vi "复材超声C扫缺陷分析评定软件-修改中.vi"() -> ()   [LabVIEW 2018]
doc: "使用该模板构建用户界面事件处理设计模式。将模板应用于对话框及其它用户界面。用户也可创建并执行VI可按照与用户界面事件相同方式处理的用户定义事件。"
uses:
  <vilib>/Utility/NIReport.llb/Report Type.ctl
  <vilib>/addons/_office/_exclsub.llb/font.ctl
  <vilib>/addons/_office/word.llb/Word Easy Table (str).vi
  <vilib>/Utility/NIReport.llb/NI_report.lvclass
  <vilib>/vision/NI_Vision_Development_Module.lvlib
  <vilib>/Utility/NIReport.llb/NI_ReportGenerationCore.lvlib
  <vilib>/addons/_office/NI_ReportGenerationToolkit.lvlib
panel:
  out "标注后的图片路径":path
  out "弥散类检测结果合并":string[][](table)
  out "分层类检测结果合并":string[][](table)
  out "反射图原始路径":path
  out "穿透图原始路径":path
  out "弥散类检测结果":string[][](table)
  out "分层类检测结果":string[][](table)
  out "部位信息":string[](array[string])=["", "34.500000", "32.500000", "1121", "34", "54.955926", "分层类", "不合格", ""]
  out "连接的字符串":string
  in  "完成标注":bool caption="定量分析"
  out "框数":dbl
  in  "Operation":enum16{"overlay rectangle"}(ring)
  out "ROI左上角坐标":cluster{i32, i32}
  out "自定义字体":T1={"Desired Font (Application)"=enum."Application Font", "[User-specified Font]"={"Font Name"="", "Size"=12, "Strikeout?"=FALSE, "Italic?"=FALSE, "Underline?"=FALSE, "Outline?"=FALSE, "Shadow?"=FALSE, "Bold?"=FALSE, "Rotation Angle"=0.0}, "Horizontal Alignment"=0, "Vertical Alignment"=0} {"Horizontal Alignment" items=["Left", "Center", "Right"]; "Vertical Alignment" items=["Bottom", "Top", "Baseline"]}
  out "标注图ROI2Mask":T2(plugin-control)
  out "透射图最大灰度值":sgl
  out "反射图最大灰度值":sgl
  out "反射图灰度表":u32[](graph)
  out "透射图灰度表":u32[](graph)
  out "总面积":i32
  out "框组":T3(array[cluster])
  out "质量等级":string
  in  "导入反射图":bool caption="导入图片"
  out "灰度阈值":dbl
  in  "stop":bool caption="停止"
  in  "导入穿透图":bool caption="导入图片"
  in  "图像预处理":bool
  in  "自定义色彩":bool
  in  "缺陷标注":bool caption="定量分析"
  in  "查看标注":bool caption="辅助定性分析"
  in  "生成评定结果":bool caption="生成原始记录"
  in  "?":enum32{"穿透图", "反射图"}(tab)
  out "穿透图":T2(plugin-control)
  out "反射图":T2(plugin-control)
  out "产品规格":cluster{"产品长度（周长）（mm）":dbl, "产品宽度（母线长）（mm）":dbl}
  out "图像分辨率":T4
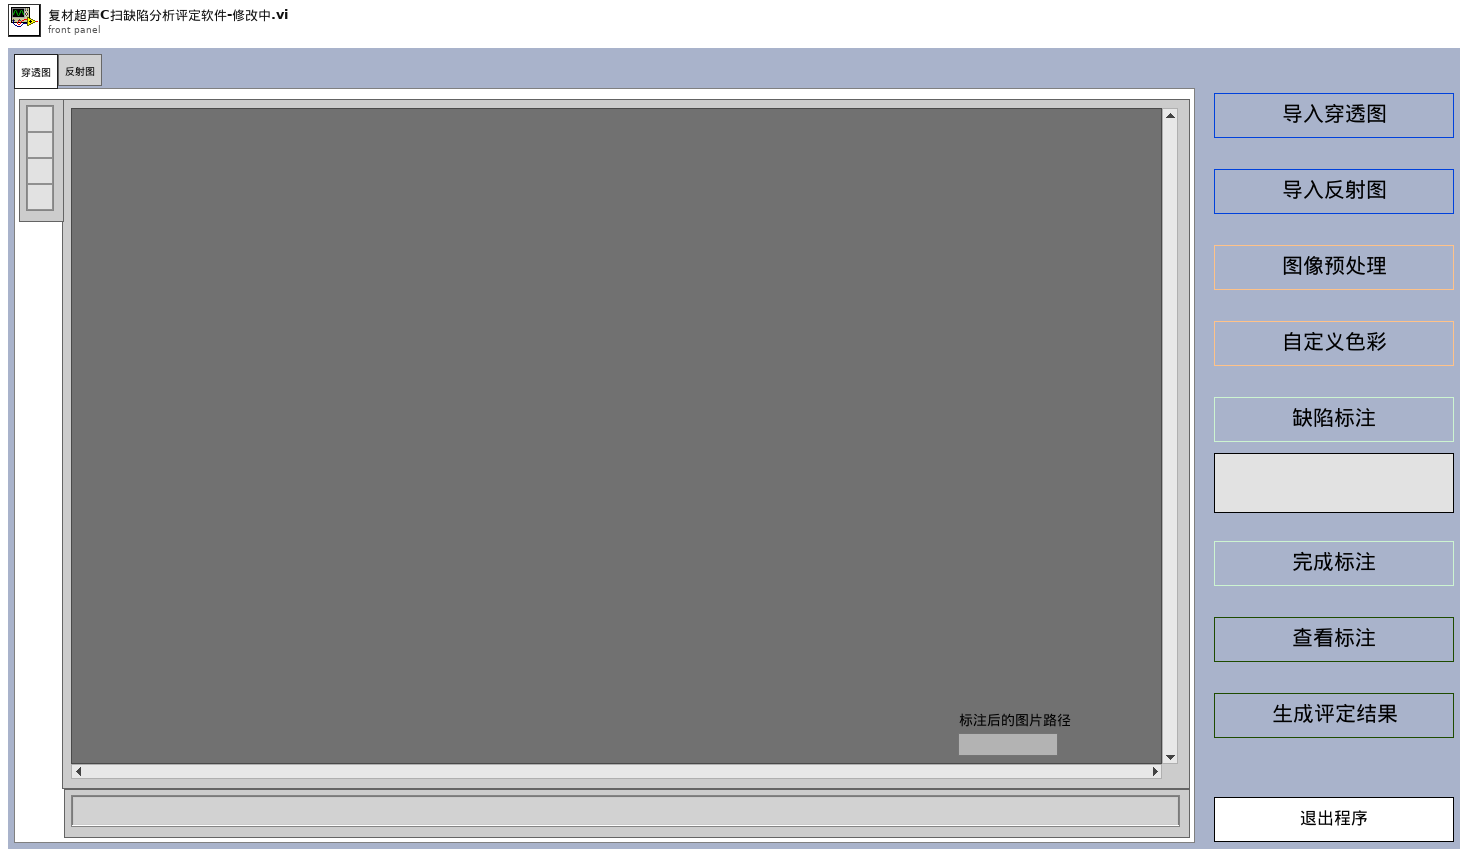
[diagram p1: front panel]
types:
  T1 = cluster{"Desired Font (Application)":enum16{"User-specified Font", "Application Font", "System Font", "Dialog Font"}, "[User-specified Font]":cluster{"Font Name":string, "Size":i16, "Strikeout?":bool, "Italic?":bool, "Underline?":bool, "Outline?":bool, "Shadow?":bool, "Bold?":bool, "Rotation Angle":dbl}, "Horizontal Alignment":i16, "Vertical Alignment":i16}
  T2 = typedef "IMAQ Image.ctl" = refnum<image>
  T3 = cluster{"Global Rectangle":i32[], "Contours":cluster{"Contour Type":u32, "ROI Type":u32, "Points":i32[]}[]}[]
  T4 = cluster{"图像X向分辨率（mm/像素）":dbl, "图像Y向分辨率（mm/像素）":dbl}
  T5 = cluster{"Zoom Tool":bool, "Selection Tool":bool, "Pan Tool":bool, "Point Tool":bool, "Line Tool":bool, "Rectangle Tool":bool, "Rotated Rectangle Tool":bool, "Polyline Tool":bool, "Polygon Tool":bool, "Freehand Tool":bool, "Closed Freehand Tool":bool, "Ellipse Tool":bool, "Annulus Tool":bool}
  T6 = enum32{"Invalid", "Standard", "Closed", "Hidden", "Minimized", "Maximized"}
  T7 = enum32{"Linear", "Log", "Exp", "Square", "Square root", "Power X", "Power 1/X"}
  T8 = enum32{"Gray", "Binary", "Gradient", "Rainbow", "Temperature"}
  T9 = typedef "NI_ReportGenerationToolkit.lvlib/font.ctl" = cluster{"font name":string, "font size":dbl, "bold":u16, "italic":u16, "underline":u16, "strike through":u16, "font color":u32}
  T10 = enum16{"maximized", "minimized", "normal", "no change"}
  T11 = typedef "NI_ReportGenerationCore.lvlib/Report Type.ctl" = enum16{"HTML", "Word", "Excel"}
  T12 = typedef "Image Type" = u32
  T13 = cluster{"Red (or Hue) value":u8, "Green (or Sat) value":u8, "Blue (or Light or Val) value":u8}[]
  T14 = cluster{"histogram":u32[], "Minimal Value":sgl, "Maximal Value":sgl, "Starting Value":sgl, "Interval Width":sgl, "Mean Value":sgl, "Standard  Variation":sgl, "Area (pixels)":i32}
  T15 = cluster{"Global Rectangle":i32[], "Contours":cluster{"Contour Type":u32, "ROI Type":u32, "Points":i32[]}[]}
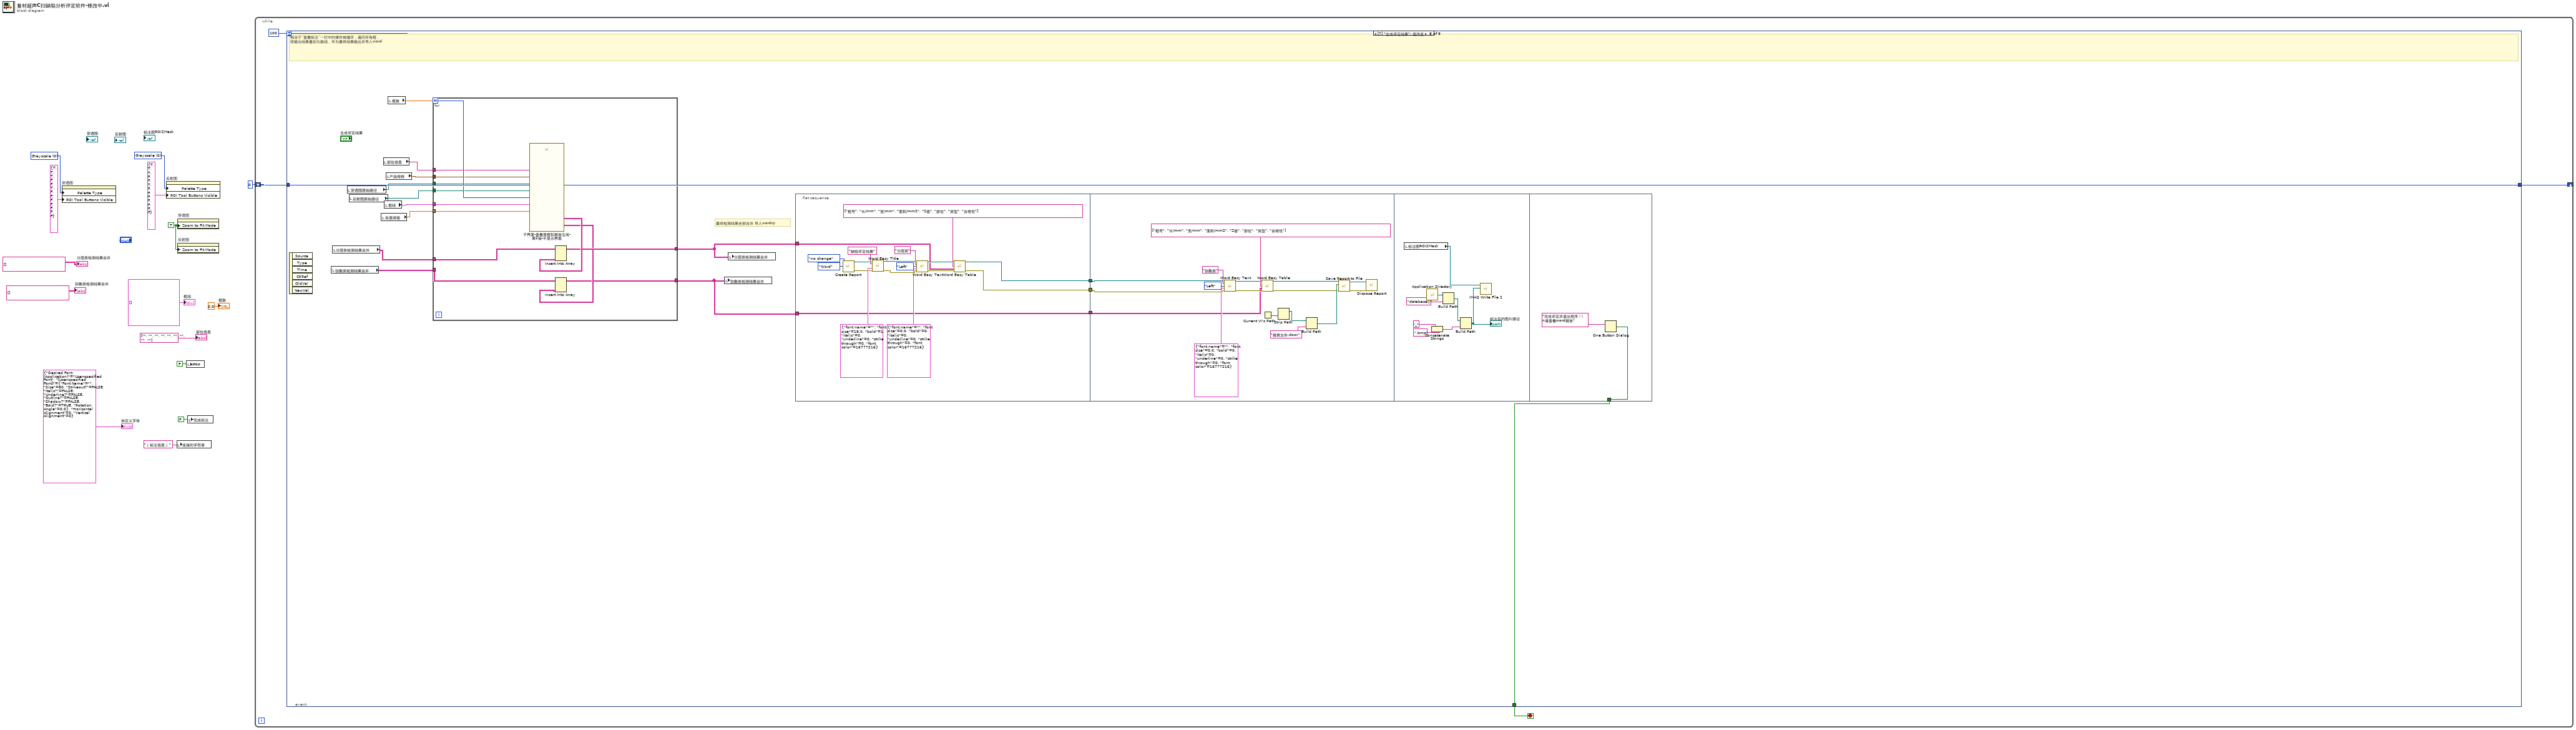
[diagram p0: block diagram]
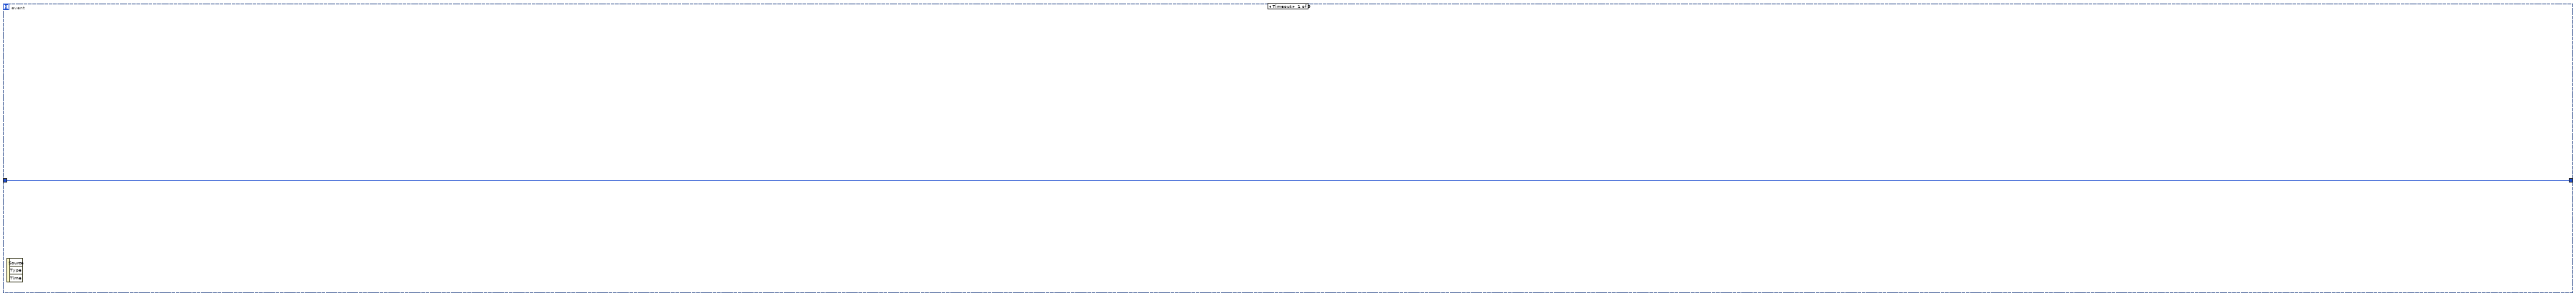
[diagram p2: hidden frame]
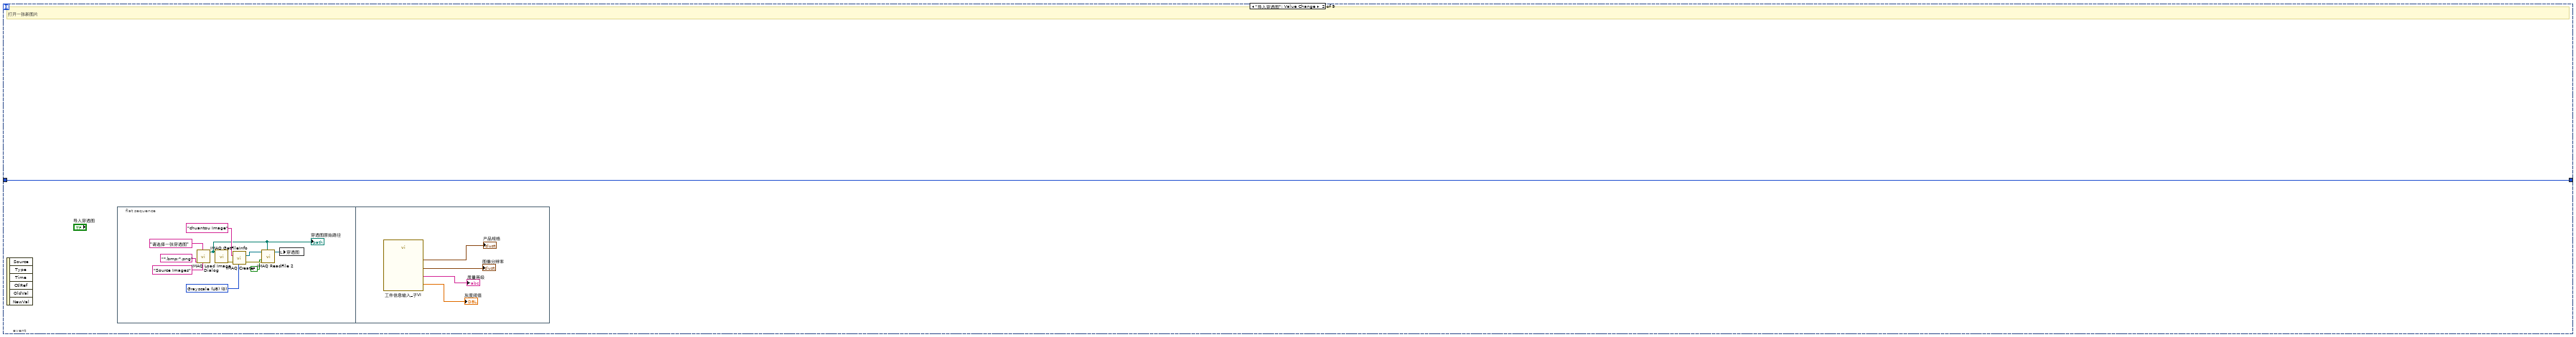
[diagram p3: hidden frame]
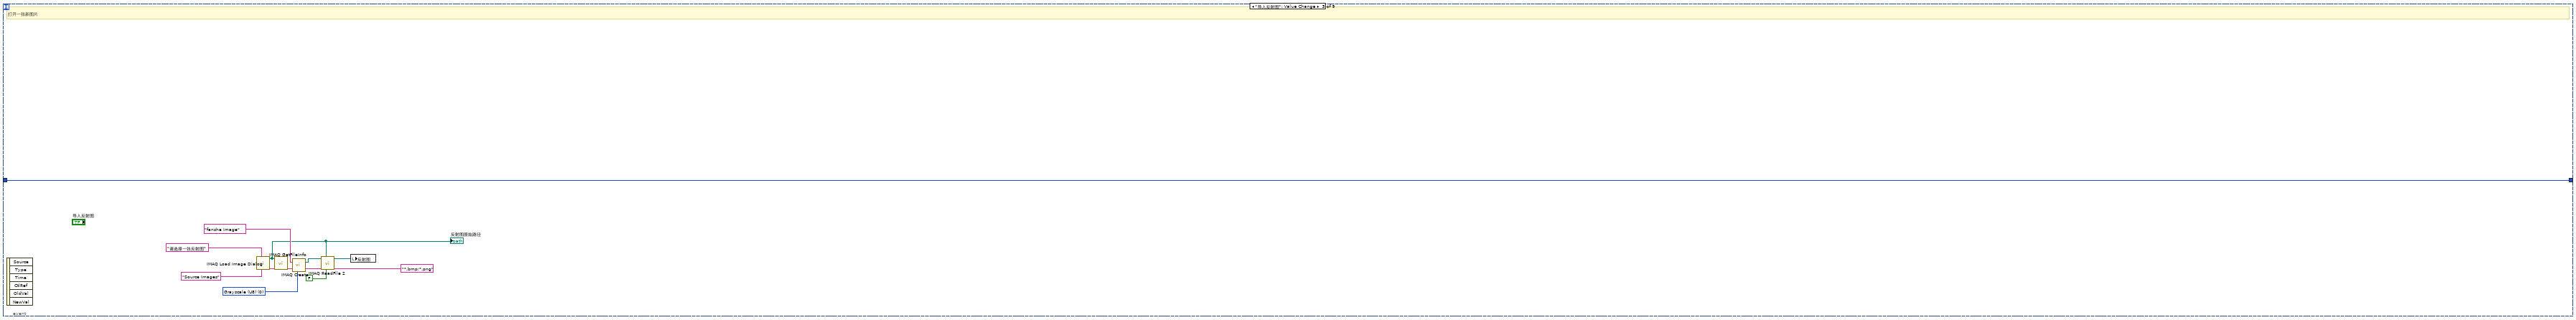
[diagram p4: hidden frame]
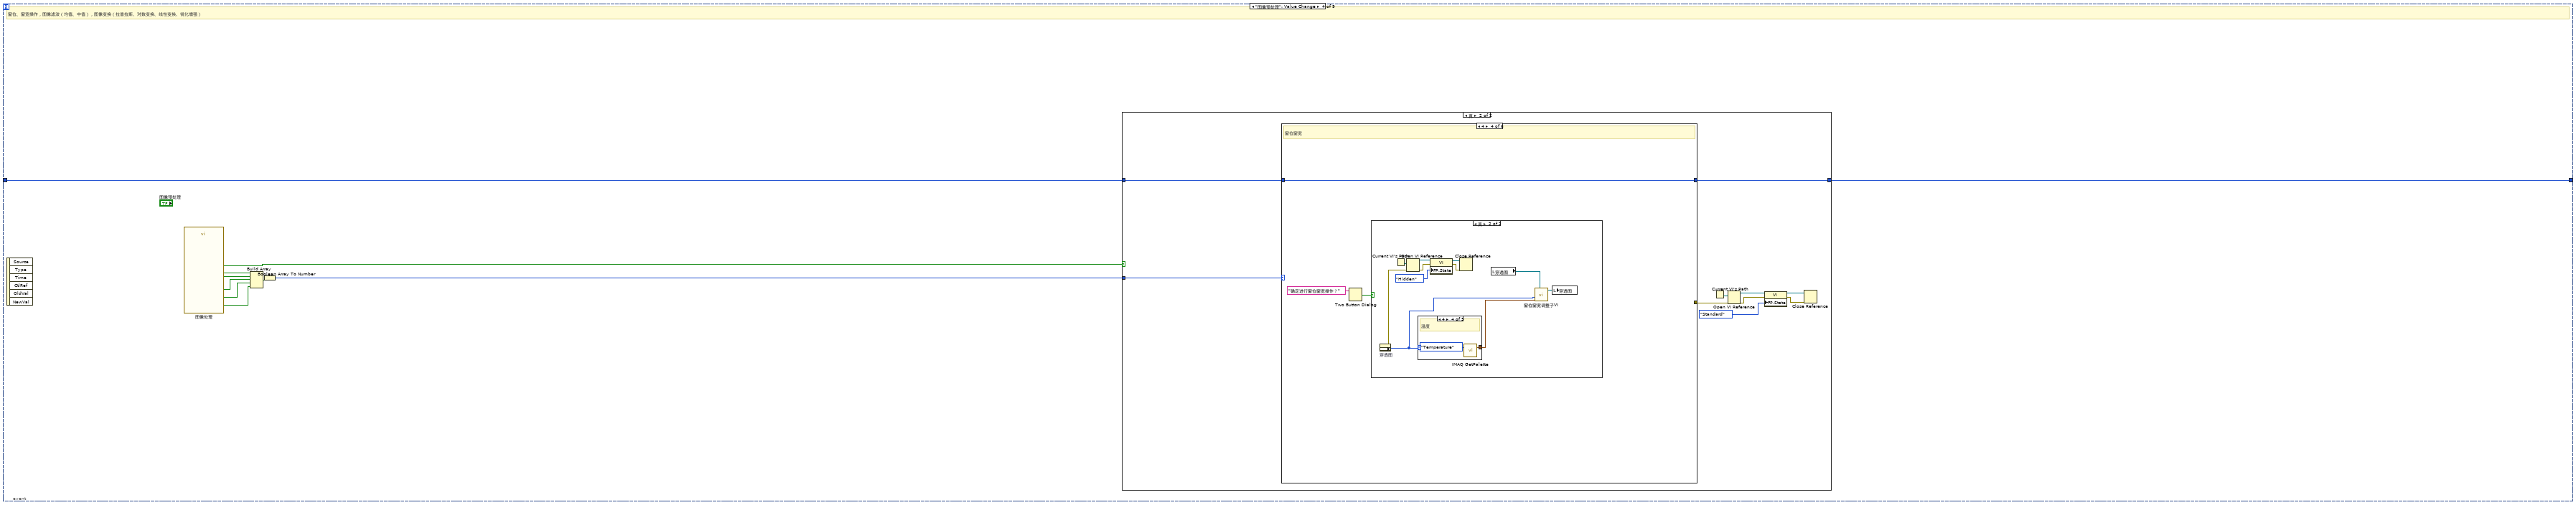
[diagram p5: hidden frame]
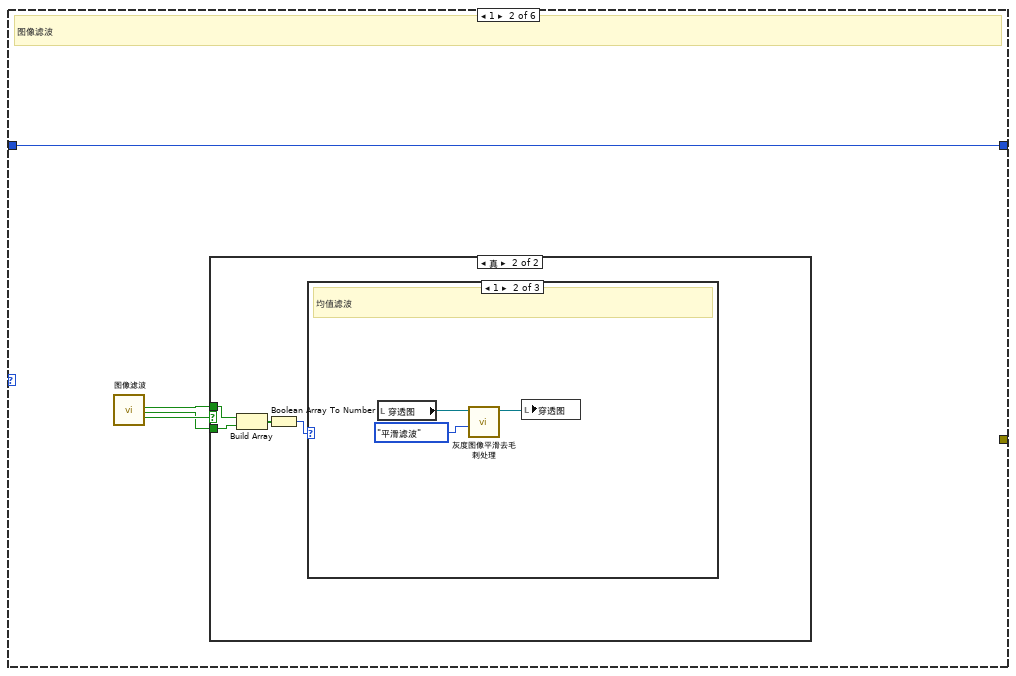
[diagram p8: hidden frame]
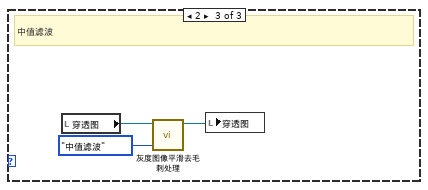
[diagram p11: hidden frame]
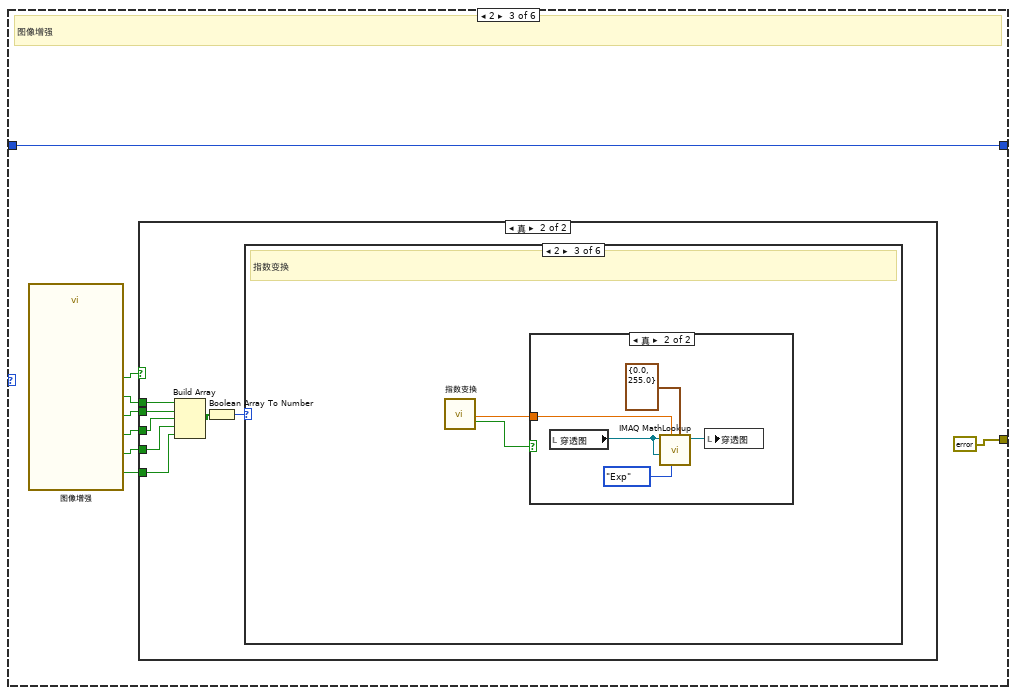
[diagram p12: hidden frame]
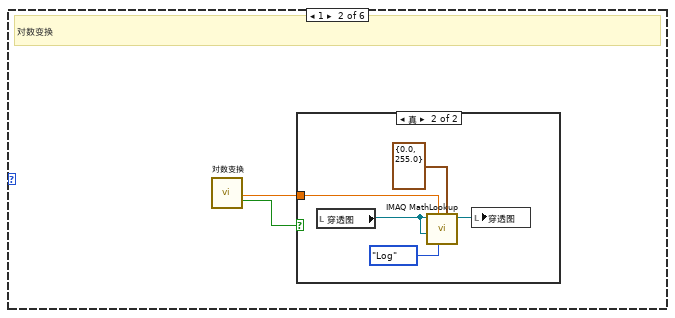
[diagram p15: hidden frame]
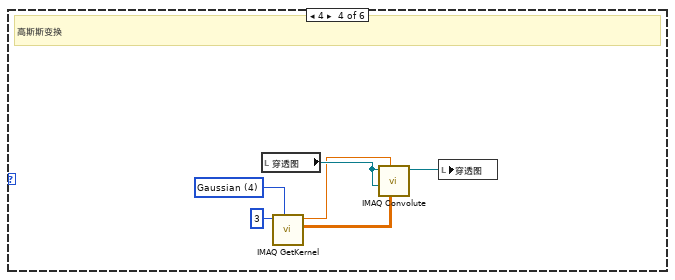
[diagram p18: hidden frame]
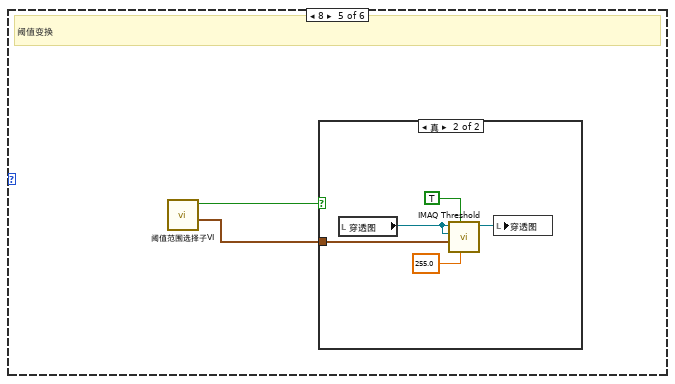
[diagram p19: hidden frame]
diagram:
  w5 = u32 0 items=["Grayscale", "Binary", "Gradient", "Rainbow", "Temperature", "User Defined", "Binary 16 Bit", "Gradient 16 Bit", "Rainbow 16 Bit", "Temperature 16 Bit", "User Defined 16 Bit"] ("Palette:Palette Type")
  w11 = TRUE ("Zoom to Fit Mode")
  w14 = u32 0 items=["Grayscale", "Binary", "Gradient", "Rainbow", "Temperature", "User Defined", "Binary 16 Bit", "Gradient 16 Bit", "Rainbow 16 Bit", "Temperature 16 Bit", "User Defined 16 Bit"] ("Palette:Palette Type")
  n1 = property on="穿透图" class="ImageControl"("Palette Type"=w14, "ROI Tool Buttons Visible"=T5 {"Zoom Tool"=TRUE, "Selection Tool"=TRUE, "Pan Tool"=TRUE, "Point Tool"=FALSE, "Line Tool"=FALSE, "Rectangle Tool"=TRUE, "Rotated Rectangle Tool"=FALSE, "Polyline Tool"=FALSE, "Polygon Tool"=FALSE, "Freehand Tool"=FALSE, "Closed Freehand Tool"=FALSE, "Ellipse Tool"=FALSE, "Annulus Tool"=FALSE} ("ROI Tool Buttons Visible:All Elements")) -> ()  [unwired: 2 in, 2 out]
  n2 = property on="反射图" class="ImageControl"("Palette Type"=w5, "ROI Tool Buttons Visible"=T5 {"Zoom Tool"=TRUE, "Selection Tool"=TRUE, "Pan Tool"=TRUE, "Point Tool"=FALSE, "Line Tool"=FALSE, "Rectangle Tool"=TRUE, "Rotated Rectangle Tool"=FALSE, "Polyline Tool"=FALSE, "Polygon Tool"=FALSE, "Freehand Tool"=FALSE, "Closed Freehand Tool"=FALSE, "Ellipse Tool"=FALSE, "Annulus Tool"=FALSE} ("ROI Tool Buttons Visible:All Elements")) -> ()  [unwired: 2 in, 2 out]
  n3 = local write "连接的字符串"("（标注信息）" ("连接的字符串")) -> ()
  n4 = property on="穿透图" class="ImageControl"("Zoom to Fit Mode"=w11) -> ()  [unwired: 2 in, 2 out]
  n5 = property on="反射图" class="ImageControl"("Zoom to Fit Mode"=w11) -> ()  [unwired: 2 in, 2 out]
  n6 = local write "stop"(FALSE ("stop")) -> ()
  n7 = local write "完成标注"(FALSE ("完成标注")) -> ()
  n8 = while {
    shift-right: [w16] -> _
    shift-left: 0 -> [w17]
    stop <- w19 stop-if-true
    n9 = event shown="[7] \"生成评定结果\": 值改变" {
      selector: _ -> [_ _ _ _ _ _ _ _ _]
      dyn-events: _ -> [_ _ _ _ _ _ _ _ _]
      timeout: 100 -> [_ _ _ _ _ _ _ _ _]
      tunnel: [_ _ _ _ _ _ _ w396 w471] -> w19
      tunnel: w17 -> [w20 w21 w48 w50 w188 _ _ w411 _]
      tunnel: [w20 w21 w48 w49 w188 _ _ w411 0] -> w16
      event Timeout {
        n10 = event-data() -> ()  [unwired: 1 in, 3 out]
      }
      event "导入穿透图": Value Change {
        # "打开一张新图片"
        n11 = event-data() -> ()  [unwired: 1 in, 6 out]
        n12 = flat-sequence {
          frame #0 {
            w24 = T12 0 items=["Grayscale (U8)", "Grayscale (I16)", "Grayscale (SGL)", "Complex (CSG)", "RGB (U32)", "HSL (U32)", "RGB (U64)", "Grayscale (U16)"] ("Image Type")
            n13 = call "IMAQ Load Image Dialog"("Pattern Label"="Source Images", "Prompt"="请选择一张穿透图" ("prompt"), "Pattern"="*.bmp;*.png") -> ("Path"=w22:path)  [unwired: 6 in, 2 out]
            "穿透图原始路径" <- w22
            n14 = call "IMAQ GetFileInfo"("File Path"=w22) -> ("error out"=w27:errorcluster)  [unwired: 4 in, 6 out]
            n15 = call "IMAQ Create"("Image Name"="chuantou Image", "Image Type"=w24, "error in (no error)"=w27) -> ("New Image"=w28:T2, "error out"=w29:errorcluster)  [unwired: 2 in]
            n16 = call "IMAQ ReadFile 2"("Use File Path Image Type"=FALSE, "File Path"=w22, "error in (no error)"=w29, "Image"=w28) -> ("Image Out"=w23:T2)  [unwired: 3 in, 4 out]
            n17 = local write "穿透图"(w23) -> ()
          }
          frame #1 {
            n18 = call "工件信息输入_子VI.vi"() -> ("质量等级"=→"质量等级":string, "灰度阈值"=→"灰度阈值":dbl, "产品规格"=→"产品规格":cluster{"产品长度（周长）（mm）":dbl, "产品宽度（母线长）（mm）":dbl}, "图像分辨率"=→"图像分辨率":T4)  [unwired: 7 in]
          }
        }
      }
      event "导入反射图": Value Change {
        w39 = T12 0 items=["Grayscale (U8)", "Grayscale (I16)", "Grayscale (SGL)", "Complex (CSG)", "RGB (U32)", "HSL (U32)", "RGB (U64)", "Grayscale (U16)"] ("Image Type")
        # "打开一张新图片"
        n19 = event-data() -> ()  [unwired: 1 in, 6 out]
        n20 = call "IMAQ Load Image Dialog"("Pattern Label"="Source Images", "Prompt"="请选择一张反射图" ("prompt"), "Pattern"="*.bmp;*.png") -> ("Path"=w37:path)  [unwired: 6 in, 2 out]
        "反射图原始路径" <- w37
        n21 = call "IMAQ GetFileInfo"("File Path"=w37) -> ("error out"=w42:errorcluster)  [unwired: 4 in, 6 out]
        n22 = call "IMAQ Create"("Image Name"="fanshe Image", "Image Type"=w39, "error in (no error)"=w42) -> ("New Image"=w43:T2, "error out"=w44:errorcluster)  [unwired: 2 in]
        n23 = call "IMAQ ReadFile 2"("Use File Path Image Type"=FALSE, "File Path"=w37, "error in (no error)"=w44, "Image"=w43) -> ("Image Out"=w38:T2)  [unwired: 3 in, 4 out]
        n24 = local write "反射图"(w38) -> ()
      }
      event "图像预处理": Value Change {
        # "窗位、窗宽操作，图像滤波（均值、中值），图像变换（拉普拉斯、对数变换、线性变换、锐化增强）"
        n25 = event-data() -> ()  [unwired: 1 in, 6 out]
        n26 = call "图像处理"() -> ("撤销图像处理"=w51:bool, "线性灰度值测量"=w52:bool, "窗位窗宽"=w57:bool, "图像增强"=w53:bool, "图像滤波"=w58:bool, "确定"=w54:bool)  [unwired: 13 in, 1 out]
        n27 = Build Array(w58, w53, w57, w52, w51) -> (w56:bool[])
        n28 = Boolean Array To Number(Boolean array=w56) -> (number=w55:u32)
        n29 = case shown="真" w54 {
          tunnel: w55 -> [_ w69]
          tunnel: w50 -> [w59 w61]
          tunnel: [w59 w60] -> w49
          frame False {
          }
          frame True {
            n30 = case shown="4" w69 {
              tunnel: [_ _ errorcluster {"status"=FALSE, "code"=0, "source"=""} ("错误输入（无错误）") _ _ _] -> w62
              tunnel: w61 -> [w70 w71 w85 w134 w157 w179]
              tunnel: [w70 w71 w85 w134 w157 w179] -> w60
              frame 0, Default {
              }
              frame 1 {
                # "图像滤波"
                n31 = call "图像滤波"() -> ("均值滤波"=w73:bool, "中值滤波"=w72:bool, "确定"=w74:bool)  [unwired: 16 in, 1 out]
                n32 = case shown="真" w74 {
                  tunnel: w73 -> [_ w77]
                  tunnel: w72 -> [_ w76]
                  frame False {
                  }
                  frame True {
                    n33 = Build Array(w77, w76) -> (w78:bool[])
                    n34 = Boolean Array To Number(Boolean array=w78) -> (number=w75:u32)
                    n35 = case shown="1" w75 {
                      frame 0, Default {
                      }
                      frame 1 {
                        # "均值滤波"
                        n36 = local read "穿透图"() -> (w81:T2)
                        n37 = call "灰度图像平滑去毛刺处理.vi"("滤波方法选择"=enum16{"中值滤波", "平滑滤波"}."平滑滤波", "Image"=w81) -> ("Image Out"=w80:T2)  [unwired: 9 in]
                        n38 = local write "穿透图"(w80) -> ()
                      }
                      frame 2 {
                        # "中值滤波"
                        n39 = local read "穿透图"() -> (w84:T2)
                        n40 = call "灰度图像平滑去毛刺处理.vi"("滤波方法选择"=enum16{"中值滤波", "平滑滤波"}."中值滤波", "Image"=w84) -> ("Image Out"=w83:T2)  [unwired: 9 in]
                        n41 = local write "穿透图"(w83) -> ()
                      }
                    }
                  }
                }
              }
              frame 2 {
                # "图像增强"
                n42 = call "图像增强"() -> ("幂变换"=w87:bool, "阈值变换"=w88:bool, "高斯变换"=w89:bool, "指数变换"=w90:bool, "对数变换"=w91:bool, "确定"=w92:bool)  [unwired: 13 in, 1 out]
                n43 = case shown="真" w92 {
                  tunnel: w91 -> [_ w97]
                  tunnel: w90 -> [_ w96]
                  tunnel: w89 -> [_ w95]
                  tunnel: w88 -> [_ w94]
                  tunnel: w87 -> [_ w93]
                  frame False {
                  }
                  frame True {
                    n44 = Build Array(w97, w96, w95, w94, w93) -> (w99:bool[])
                    n45 = Boolean Array To Number(Boolean array=w99) -> (number=w98:u32)
                    n46 = case shown="2" w98 {
                      frame 0, Default {
                      }
                      frame 1 {
                        # "对数变换"
                        n47 = call "对数变换"() -> ("变换系数K"=w100:dbl, "确定"=w101:bool)  [unwired: 17 in, 1 out]
                        n48 = case shown="真" w101 {
                          tunnel: w100 -> [_ w102]
                          frame False {
                          }
                          frame True {
                            n49 = local read "穿透图"() -> (w106:T2)
                            n50 = call "IMAQ MathLookup"("Range"=cluster{"Minimum":sgl, "Maximum":sgl} {"Minimum"=0.0, "Maximum"=255.0}, "Operator"=T7."Log", "X Value"=w102, "Image Dst"=w106, "Image Src"=w106) -> ("Image Dst Out"=w104:T2)  [unwired: 5 in, 1 out]
                            n51 = local write "穿透图"(w104) -> ()
                          }
                        }
                      }
                      frame 2 {
                        # "指数变换"
                        n52 = call "指数变换"() -> ("变换系数K"=w107:dbl, "确定"=w108:bool)  [unwired: 17 in, 1 out]
                        n53 = case shown="真" w108 {
                          tunnel: w107 -> [_ w109]
                          frame False {
                          }
                          frame True {
                            n54 = local read "穿透图"() -> (w113:T2)
                            n55 = call "IMAQ MathLookup"("Range"=cluster{"Minimum":sgl, "Maximum":sgl} {"Minimum"=0.0, "Maximum"=255.0}, "Operator"=T7."Exp", "X Value"=w109, "Image Dst"=w113, "Image Src"=w113) -> ("Image Dst Out"=w111:T2)  [unwired: 5 in, 1 out]
                            n56 = local write "穿透图"(w111) -> ()
                          }
                        }
                      }
                      frame 4 {
                        w119 = u16 4 items=["Gradient"=1, "Laplacian"=2, "Smoothing"=3, "Gaussian"=4] ("Kernel Family")
                        # "高斯斯变换"
                        n57 = local read "穿透图"() -> (w116:T2)
                        n58 = call "IMAQ GetKernel"("Kernel Family"=w119, "Kernel Size (3,5,...)"=3) -> ("Kernel"=w117:sgl[][], "Divider"=w114:sgl)  [unwired: 6 in, 2 out]
                        n59 = call "IMAQ Convolute"("Kernel"=w117, "Divider (kernel sum)"=w114, "Image Dst"=w116, "Image Src"=w116) -> ("Image Dst Out"=w115:T2)  [unwired: 6 in, 1 out]
                        n60 = local write "穿透图"(w115) -> ()
                      }
                      frame 8 {
                        # "阈值变换"
                        n61 = call "阈值范围选择子VI.vi"() -> ("阈值范围"=w120:cluster{"Lower value":sgl, "Upper value":sgl}, "确定执行"=w121:bool)  [unwired: 10 in]
                        n62 = case shown="真" w121 {
                          tunnel: w120 -> [_ w123]
                          frame False {
                          }
                          frame True {
                            n63 = local read "穿透图"() -> (w126:T2)
                            n64 = call "IMAQ Threshold"("Replace Value"=sgl 255.0, "Keep/Replace Value (Replace)"=TRUE, "Range"=w123, "Image Dst"=w126, "Image Src"=w126) -> ("Image Dst Out"=w125:T2)  [unwired: 5 in, 1 out]
                            n65 = local write "穿透图"(w125) -> ()
                          }
                        }
                      }
                      frame 16 {
                        # "幂变换"
                        n66 = call "幂变换"() -> ("变换系数K"=w127:dbl, "确定"=w128:bool)  [unwired: 17 in, 1 out]
                        n67 = case shown="真" w128 {
                          tunnel: w127 -> [_ w129]
                          frame False {
                          }
                          frame True {
                            n68 = local read "穿透图"() -> (w133:T2)
                            n69 = call "IMAQ MathLookup"("Range"=cluster{"Minimum":sgl, "Maximum":sgl} {"Minimum"=0.0, "Maximum"=255.0}, "Operator"=T7."Power 1/X", "X Value"=w129, "Image Dst"=w133, "Image Src"=w133) -> ("Image Dst Out"=w131:T2)  [unwired: 5 in, 1 out]
                            n70 = local write "穿透图"(w131) -> ()
                          }
                        }
                      }
                    }
                  }
                }
              }
              frame 4 {
                # "窗位窗宽"
                n71 = Two Button Dialog(message="确定进行窗位窗宽操作？" ("消息")) -> (T button?=w136:bool)  [unwired: 2 in]
                n72 = case shown="真" w136 {
                  frame False {
                  }
                  frame True {
                    n73 = property on="穿透图" class="ImageControl"() -> (error out=w138:errorcluster, "Palette Type"=w145:u32)  [unwired: 2 in, 1 out]
                    n74 = Current VI's Path() -> (path=w140:path)
                    n75 = Open VI Reference(vi path=w140, error in (no error)=w138) -> (vi reference=w141:refnum<vi>, error out=w143:errorcluster)  [unwired: 4 in]
                    n76 = case shown="4" w145 {
                      tunnel: [w148 w150 w152 w154 w156] -> w146
                      frame 0, Default {
                        # "灰度"
                        n77 = call "IMAQ GetPalette"("Palette Number (gray)"=T8."Gray") -> ("Color Palette"=w148:cluster{"Red":u8, "Green":u8, "Blue":u8}[])  [unwired: 4 in, 1 out]
                      }
                      frame 2 {
                        # "梯度"
                        n78 = call "IMAQ GetPalette"("Palette Number (gray)"=T8."Gradient") -> ("Color Palette"=w150:cluster{"Red":u8, "Green":u8, "Blue":u8}[])  [unwired: 4 in, 1 out]
                      }
                      frame 3 {
                        # "彩虹"
                        n79 = call "IMAQ GetPalette"("Palette Number (gray)"=T8."Rainbow") -> ("Color Palette"=w152:cluster{"Red":u8, "Green":u8, "Blue":u8}[])  [unwired: 4 in, 1 out]
                      }
                      frame 4 {
                        # "温度"
                        n80 = call "IMAQ GetPalette"("Palette Number (gray)"=T8."Temperature") -> ("Color Palette"=w154:cluster{"Red":u8, "Green":u8, "Blue":u8}[])  [unwired: 4 in, 1 out]
                      }
                      frame 5 {
                        # "自定义"
                        n81 = property on="穿透图" class="ImageControl"() -> ("User Palette"=w156:cluster{"Red":u8, "Green":u8, "Blue":u8}[])  [unwired: 2 in, 2 out]
                      }
                    }
                    n82 = property class="VI"(reference=w141, error in=w143, "FP.State"=T6."Hidden" ("前面板窗口:状态")) -> (reference out=w142:refnum<vi>, error out=w144:errorcluster)
                    n83 = Close Reference(reference=w142, error in (no error)=w144) -> ()  [unwired: 1 out]
                    n84 = local read "穿透图"() -> (w137:T2)
                    n85 = call "窗位窗宽调整子VI.vi"("Image in"=w137, "Palette:User Palette"=w146, "Palette:Palette Type"=w145) -> ("Image out"=w147:T2)  [unwired: 8 in]
                    n86 = local write "穿透图"(w147) -> ()
                  }
                }
              }
              frame 8 {
                # "查看线灰度值曲线，用于精确测量"
                n87 = Current VI's Path() -> (path=w164:path)
                n88 = Open VI Reference(vi path=w164) -> (vi reference=w163:refnum<vi>, error out=w161:errorcluster)  [unwired: 5 in]
                n89 = property class="VI"(reference=w163, error in=w161, "FP.State"=T6."Hidden" ("前面板窗口:状态")) -> (reference out=w162:refnum<vi>, error out=w160:errorcluster)
                n90 = Close Reference(reference=w162, error in (no error)=w160) -> (error out=w158:errorcluster)
                n91 = case shown="无错误" w158 {
                  frame No Error {
                    n92 = property on="穿透图" class="ImageControl"() -> ("Palette Type"=w166:u32)  [unwired: 2 in, 2 out]
                    n93 = case shown="2" w166 {
                      tunnel: [w169 w171 w173 w175 w177] -> w165
                      frame 0, Default {
                        # "灰度"
                        n94 = call "IMAQ GetPalette"("Palette Number (gray)"=T8."Gray") -> ("Color Palette"=w169:cluster{"Red":u8, "Green":u8, "Blue":u8}[])  [unwired: 4 in, 1 out]
                      }
                      frame 2 {
                        # "梯度"
                        n95 = call "IMAQ GetPalette"("Palette Number (gray)"=T8."Gradient") -> ("Color Palette"=w171:cluster{"Red":u8, "Green":u8, "Blue":u8}[])  [unwired: 4 in, 1 out]
                      }
                      frame 3 {
                        # "彩虹"
                        n96 = call "IMAQ GetPalette"("Palette Number (gray)"=T8."Rainbow") -> ("Color Palette"=w173:cluster{"Red":u8, "Green":u8, "Blue":u8}[])  [unwired: 4 in, 1 out]
                      }
                      frame 4 {
                        # "温度"
                        n97 = call "IMAQ GetPalette"("Palette Number (gray)"=T8."Temperature") -> ("Color Palette"=w175:cluster{"Red":u8, "Green":u8, "Blue":u8}[])  [unwired: 4 in, 1 out]
                      }
                      frame 5 {
                        # "自定义"
                        n98 = property on="穿透图" class="ImageControl"() -> ("User Palette"=w177:cluster{"Red":u8, "Green":u8, "Blue":u8}[])  [unwired: 2 in, 2 out]
                      }
                    }
                    n99 = local read "穿透图"() -> (w168:T2)
                    n100 = local read "图像分辨率"() -> (w167:T4)
                    n101 = call "线性灰度值曲线查看子VI.vi"("Palette:User Palette"=w165, "图像分辨率"=w167, "Image"=w168) -> ()  [unwired: 9 in]
                  }
                  frame Error {
                  }
                }
              }
              frame 16 {
                # "撤销图像处理，恢复原图"
                n102 = call "IMAQ Create"("Image Name"="P1") -> ("New Image"=w178:T2)  [unwired: 4 in, 1 out]
                n103 = local write "穿透图"(w178) -> ()
              }
            }
            n104 = Current VI's Path() -> (path=w68:path)
            n105 = Open VI Reference(vi path=w68, error in (no error)=w62) -> (vi reference=w67:refnum<vi>, error out=w64:errorcluster)  [unwired: 4 in]
            n106 = property class="VI"(reference=w67, error in=w64, "FP.State"=T6."Standard" ("前面板窗口:状态")) -> (reference out=w65:refnum<vi>, error out=w63:errorcluster)
            n107 = Close Reference(reference=w65, error in (no error)=w63) -> ()  [unwired: 1 out]
          }
        }
      }
      event "自定义色彩": Value Change {
        # "色彩、色阶自定义"
        n108 = event-data() -> ()  [unwired: 1 in, 6 out]
        n109 = call "调色板"() -> ("自定义显示"=w182:bool, "温度显示"=w183:bool, "彩虹显示"=w184:bool, "梯度显示"=w185:bool, "灰度显示"=w186:bool, "确定"=w187:bool)  [unwired: 13 in, 1 out]
        n110 = Build Array(w186, w185, w184, w183, w182) -> (w181:bool[])
        n111 = case shown="假" w187 {
          tunnel: w181 -> [_ w191]
          frame False {
          }
          frame True {
            n112 = Boolean Array To Number(Boolean array=w191) -> (number=w190:u32)
            n113 = case shown="16" w190 {
              tunnel: [w192 w193 w194 w195 w196 w198] -> w189
              frame 0, Default {
                w192 = u32 0 items=["Grayscale", "Binary", "Gradient", "Rainbow", "Temperature", "User Defined", "Binary 16 Bit", "Gradient 16 Bit", "Rainbow 16 Bit", "Temperature 16 Bit", "User Defined 16 Bit"] ("Palette:Palette Type")
              }
              frame 1 {
                w193 = u32 0 items=["Grayscale", "Binary", "Gradient", "Rainbow", "Temperature", "User Defined", "Binary 16 Bit", "Gradient 16 Bit", "Rainbow 16 Bit", "Temperature 16 Bit", "User Defined 16 Bit"] ("Palette:Palette Type")
                # "灰度"
              }
              frame 2 {
                w194 = u32 2 items=["Grayscale", "Binary", "Gradient", "Rainbow", "Temperature", "User Defined", "Binary 16 Bit", "Gradient 16 Bit", "Rainbow 16 Bit", "Temperature 16 Bit", "User Defined 16 Bit"] ("Palette:Palette Type")
                # "梯度"
              }
              frame 4 {
                w195 = u32 3 items=["Grayscale", "Binary", "Gradient", "Rainbow", "Temperature", "User Defined", "Binary 16 Bit", "Gradient 16 Bit", "Rainbow 16 Bit", "Temperature 16 Bit", "User Defined 16 Bit"] ("Palette:Palette Type")
                # "彩虹"
              }
              frame 8 {
                w196 = u32 4 items=["Grayscale", "Binary", "Gradient", "Rainbow", "Temperature", "User Defined", "Binary 16 Bit", "Gradient 16 Bit", "Rainbow 16 Bit", "Temperature 16 Bit", "User Defined 16 Bit"] ("Palette:Palette Type")
                # "温度"
              }
              frame 16 {
                w198 = u32 5 items=["Grayscale", "Binary", "Gradient", "Rainbow", "Temperature", "User Defined", "Binary 16 Bit", "Gradient 16 Bit", "Rainbow 16 Bit", "Temperature 16 Bit", "User Defined 16 Bit"] ("Palette:Palette Type")
                # "自定义"
                n114 = call "自定义成像色谱20200214.vi"() -> ("Color palette"=w197:T13)  [unwired: 8 in, 1 out]
                n115 = property on="穿透图" class="ImageControl"("User Palette"=w197) -> ()  [unwired: 2 in, 2 out]
              }
            }
            n116 = property on="穿透图" class="ImageControl"("Palette Type"=w189) -> ()  [unwired: 2 in, 2 out]
          }
        }
      }
      event "缺陷标注": Value Change {
        # "手动画框ROI，提取框组（坐标）、框数等信息 \n并同时也要进行阈值分割、缺陷特征提取 \n有关数据将存储并用于后续的生成评定结果"
        n117 = event-data() -> ()  [unwired: 1 in, 6 out]
        n118 = One Button Dialog(message="开始标注！\n全部标注完成后，\n请点击“完成标注”按钮" ("消息")) -> ()  [unwired: 1 in, 1 out]
        n119 = while {
          shift-right: [w223] -> _
          shift-left: _ -> [w222]
          tunnel: [w208] -> _
          tunnel: [w207] -> _
          stop <- w204 stop-if-true
          (unwired) "_" ("名称或相对路径")
          (unwired) ".docx" ("名称或相对路径")
          w206 = i32[] [2] items=["No Event"=0, "Click Event"=1, "Draw Event"=2, "Size Event"=4, "Scroll Event"=5, "Double Click Event"=8] ("Which Events")
          # "循环的方式给输入图像手动画框"
          n120 = local read "穿透图"() -> (w212:T2)
          n121 = local read "反射图"() -> (w213:T2)
          n122 = invoke on="穿透图" class="ImageControl" method="Get Last Event"("Which Events"=w206) -> ("Type"=w205:i32)  [unwired: 7 in, 7 out]
          n123 = call "IMAQ Histogram"("Number of Classes"=256, "Interval Range"=cluster{"Minimum":sgl, "Maximum":sgl} {"Minimum"=0.0, "Maximum"=255.0}, "Image"=w213) -> ("Histogram Report"=w215:T14)  [unwired: 7 in, 1 out]
          n124 = call "IMAQ Histogram"("Number of Classes"=256, "Interval Range"=cluster{"Minimum":sgl, "Maximum":sgl} {"Minimum"=0.0, "Maximum"=255.0}, "Image"=w212) -> ("Histogram Report"=w217:T14)  [unwired: 7 in, 1 out]
          n125 = Unbundle(w215) -> ("histogram"=→"反射图灰度表":u32[], "Maximal Value"=→"反射图最大灰度值":sgl)  [unwired: 6 out]
          n126 = Unbundle(w217) -> ("histogram"=→"透射图灰度表":u32[], "Maximal Value"=→"透射图最大灰度值":sgl, "Area (pixels)"=→"总面积":i32)  [unwired: 5 out]
          n127 = Not Equal To 0?(x=w205) -> (x != 0?=w224:bool)
          n128 = case shown="真" w224 {
            tunnel: w212 -> [w263 w271]
            tunnel: [w263 w270] -> w208
            tunnel: "Operation" -> [_ w269]
            tunnel: [w261 w264] -> w223
            tunnel: w222 -> [w261 w268]
            tunnel: w213 -> [w260 w267]
            tunnel: [w260 w266] -> w207
            frame False {
              n129 = Wait (ms)(milliseconds to wait=u32 50) -> ()  [unwired: 1 out]
            }
            frame True {
              n130 = property on="穿透图" class="ImageControl"() -> ("ROI"=w265:T15)  [unwired: 2 in, 2 out]
              n131 = case shown="\"overlay rectangle\"" w269 {
                tunnel: w271 -> [w290]
                tunnel: w265 -> [w288]
                tunnel: [w289] -> w270
                tunnel: w268 -> [w287]
                tunnel: w267 -> [w286]
                tunnel: [w285] -> w266
                tunnel: [w284] -> w264
                frame "overlay rectangle" {
                  n132 = flat-sequence {
                    tunnel: w290 -> [w292]
                    tunnel: [w292] -> w283
                    tunnel: w288 -> [w295]
                    tunnel: [w295] -> w282
                    tunnel: w287 -> [w294]
                    tunnel: w286 -> [w291]
                    tunnel: [w291] -> w281
                    tunnel: [w293] -> w280
                    tunnel: w283 -> [w304]
                    tunnel: w282 -> [w303]
                    tunnel: w281 -> [w309]
                    tunnel: w280 -> [w301]
                    tunnel: [w310] -> w279
                    tunnel: [w308] -> w278
                    tunnel: [w301] -> w277
                    tunnel: [w298] -> w276
                    tunnel: [w296] -> w272
                    tunnel: w279 -> [w334]
                    tunnel: w278 -> [w333]
                    tunnel: w277 -> [w332]
                    tunnel: w276 -> [w323]
                    tunnel: [w334] -> w275
                    tunnel: [w333] -> w274
                    tunnel: [w332] -> w273
                    tunnel: w272 -> [w319]
                    tunnel: [w341] -> w284
                    tunnel: [w342] -> w285
                    tunnel: [w343] -> w289
                    tunnel: w275 -> [w343]
                    tunnel: w274 -> [w342]
                    tunnel: w273 -> [w341]
                    frame #0 {
                      # "将当前ROI数据存入框组内"
                      n133 = Build Array (concatenate)(w294, w295) -> (w293:T3)
                      n134 = local write "框组"(w293) -> ()
                    }
                    frame #1 {
                      w306 = u32[] [0] ("Colors (Green)")
                      w302 = u32 16711776 ("Text Color (black)")
                      # "在反射图上对应位置画框"
                      # "在穿透图上画框"
                      # "图层名Group与“框&图层计数”变量同名，\neg：1号框对应group1"
                      # "overlay text在ROI的左上角添加计数显示"
                      # "overlay ROI代表用户手画绿色框的图层添加"
                      n135 = Unbundle(w303) -> ("Global Rectangle"=w316:i32[])  [unwired: 1 out]
                      n136 = local read "框组"() -> (w313:T3)
                      n137 = Index Array(array=w316, index=0 ("索引")) -> (element=w315:i32)
                      n138 = Index Array(array=w316, index=1 ("索引")) -> (element=w314:i32)
                      n139 = Array Size(array=w313) -> (size(s)=w296:i32)
                      n140 = Bundle(w315, w314) -> (w305:cluster{i32, i32})  [unwired: 1 in]
                      "ROI左上角坐标" <- w305
                      n141 = Number To Decimal String(number=w296) -> (decimal integer string=w297:string)  [unwired: 1 in]
                      n142 = Concatenate Strings(w297, "#" ("字符串")) -> (w298:string)
                      n143 = call "IMAQ Overlay ROI"("Colors (Green)"=w306, "Group"=w298, "ROI Descriptor"=w303, "Image"=w304) -> ("Image Out"=w317:T2)  [unwired: 6 in, 1 out]
                      n144 = call "IMAQ Overlay ROI"("Colors (Green)"=w306, "Group"=w298, "ROI Descriptor"=w303, "Image"=w309) -> ("Image Out"=w307:T2)  [unwired: 6 in, 1 out]
                      n145 = local write "框数"(w296) -> ()
                      n146 = local read "自定义字体"() -> (w300:T1)
                      n147 = call "IMAQ Overlay Text"("Group"=w298, "Text Color (black)"=w302, "Font, Size & Style"=w300, "String"=w298, "Origin"=w305, "Image"=w317) -> ("Image Out"=w310:T2)  [unwired: 4 in, 1 out]
                      n148 = call "IMAQ Overlay Text"("Group"=w298, "Text Color (black)"=w302, "Font, Size & Style"=w300, "String"=w298, "Origin"=w305, "Image"=w307) -> ("Image Out"=w308:T2)  [unwired: 4 in, 1 out]
                    }
                    frame #2 {
                      # "存放部位信息的1D数组，后续生成报告使用"
                      # "0：位于蒙皮部位\n1：位于筋条部位"
                      n149 = call "缺陷部位标注"() -> ("位于筋条处"=w328:bool, "位于蒙皮处"=w327:bool)  [unwired: 16 in, 2 out]
                      n150 = Decrement(x=w319) -> (x-1=w318:i32)
                      n151 = local read "部位信息"() -> (w322:string[])
                      n152 = Build Array(w327, w328) -> (w329:bool[])
                      n153 = Boolean Array To Number(Boolean array=w329) -> (number=w330:u32)
                      n154 = case shown="1, 默认" w330 {
                        tunnel: ["蒙皮处" ("t") "筋条处" ("t")] -> w321
                        frame 1, Default {
                        }
                        frame 2 {
                        }
                      }
                      n155 = Concatenate Strings("框号为" ("字符串"), w323, "\n", "类别为" ("字符串"), w321) -> (→"连接的字符串":string)
                      n156 = Insert Into Array(array=w322, index=w318, new element=w321) -> (w320:string[])
                      n157 = local write "部位信息"(w320) -> ()
                    }
                    frame #3 {
                      n158 = Two Button Dialog(message="是否需要删除标注" ("消息"), 1:"是" ("F按钮名称（“取消”）"), 2:"否" ("T按钮名称（“确定”）")) -> (T button?=w339:bool)
                      n159 = case shown="假" w339 {
                        frame False {
                          n160 = call "用户输入"() -> ("框号"=w344:dbl, "确定"=w345:bool)  [unwired: 17 in, 1 out]
                          n161 = case shown="真" w345 {
                            tunnel: w344 -> [_ w346]
                            frame False {
                              # "用户取消操作"
                            }
                            frame True {
                              n162 = stacked-sequence {
                                tunnel: w346 -> [_ w354 _]
                                frame #0 {
                                # "1. 删除所有框"
                                n163 = local read "反射图"() -> (w348:T2)
                                n164 = local read "穿透图"() -> (w347:T2)
                                n165 = call "IMAQ Clear Overlay"("Image"=w348) -> ()  [unwired: 9 in, 2 out]
                                n166 = call "IMAQ Clear Overlay"("Image"=w347) -> ()  [unwired: 9 in, 2 out]
                                }
                                frame #1 {
                                # "2. 删除框组中指定元素"
                                n167 = local read "部位信息"() -> (w351:string[])
                                n168 = local read "框组"() -> (w353:T3)
                                n169 = Decrement(x=w354) -> (x-1=w350:dbl)
                                n170 = Delete From Array(array=w351, index=w350) -> (array with subset deleted=w349:string[])  [unwired: 1 in, 1 out]
                                n171 = Delete From Array(array=w353, index=w350) -> (array with subset deleted=w352:T3)  [unwired: 1 in, 1 out]
                                n172 = local write "框组"(w352) -> ()
                                n173 = local write "部位信息"(w349) -> ()
                                }
                                frame #2 {
                                # "3. 重画所有框"
                                n174 = while {
                                i -> [w369]
                                stop <- w358 stop-if-true
                                n175 = local read "框组"() -> (w362:T3)
                                n176 = local read "穿透图"() -> (w368:T2)
                                n177 = local read "反射图"() -> (w363:T2)
                                n178 = Array Size(array=w362) -> (size(s)=w365:i32)
                                n179 = Index Array(array=w362, index=w369) -> (element=w357:T15)
                                n180 = Increment(x=w369) -> (x+1=w378:i32)
                                n181 = Unbundle(w357) -> ("Global Rectangle"=w366:i32[])  [unwired: 1 out]
                                n182 = call "IMAQ Overlay ROI"("ROI Descriptor"=w357, "Image"=w368) -> ("Image Out"=w376:T2)  [unwired: 8 in, 1 out]
                                n183 = call "IMAQ Overlay ROI"("ROI Descriptor"=w357, "Image"=w363) -> ("Image Out"=w371:T2)  [unwired: 8 in, 1 out]
                                n184 = Greater Or Equal?(x=w378, y=w365) -> (x >= y?=w358:bool)
                                n185 = local read "自定义字体"() -> (w356:T1)
                                n186 = Index Array(array=w366, index=1 ("索引")) -> (element=w374:i32)
                                n187 = Index Array(array=w366, index=0 ("索引")) -> (element=w373:i32)
                                n188 = Bundle(w373, w374) -> (w360:cluster{i32, i32})  [unwired: 1 in]
                                n189 = Number To Decimal String(number=w378) -> (decimal integer string=w359:string)  [unwired: 1 in]
                                n190 = Concatenate Strings(w359, "#" ("字符串")) -> (w355:string)
                                n191 = call "IMAQ Overlay Text"("Text Color (black)"=u32 16711680, "Font, Size & Style"=w356, "String"=w355, "Origin"=w360, "Image"=w371) -> ("Image Out"=w364:T2)  [unwired: 5 in, 1 out]
                                n192 = call "IMAQ Overlay Text"("Text Color (black)"=u32 16711680, "Font, Size & Style"=w356, "String"=w355, "Origin"=w360, "Image"=w376) -> ("Image Out"=w367:T2)  [unwired: 5 in, 1 out]
                                n193 = local write "反射图"(w364) -> ()
                                n194 = local write "穿透图"(w367) -> ()
                                n195 = local write "框数"(w365) -> ()
                                }
                                }
                              }
                            }
                          }
                        }
                        frame True {
                        }
                      }
                    }
                  }
                }
              }
            }
          }
          n196 = case shown="真" "完成标注" {
            tunnel: [FALSE ("T button?") w228] -> w202
            frame False {
            }
            frame True {
              n197 = Two Button Dialog(message="请确认是否完成标注" ("消息")) -> (T button?=w228:bool)  [unwired: 2 in]
            }
          }
          n198 = case shown="真" w202 {
            tunnel: [FALSE w230] -> w201
            frame False {
            }
            frame True {
              n199 = while {
                tunnel: [w235] -> w230
                i -> [w241]
                stop <- w235 stop-if-true
                w246 = 2 items=["White", "Black", "Inverted", "Black on White", "White on Black"] ("Color")
                w250 = u16 2 items=["Frame", "Paint", "Invert Frame", "Invert Paint"] ("Draw Mode")
                w243 = u16 1 items=["Line", "Rectangle", "Oval"] ("Shape to draw")
                # "生成绘制了ROI的图像\n可以用于后续的图片导出保存"
                n200 = local read "框组"() -> (w240:T3)
                n201 = local read "穿透图"() -> (w237:T2)
                n202 = local read "标注图ROI2Mask"() -> (w236:T2)
                n203 = Array Size(array=w240) -> (size(s)=w258:i32)
                n204 = Index Array(array=w240, index=w241) -> (element=w239:T15)
                n205 = Unbundle(w239) -> ("Global Rectangle"=w238:i32[])  [unwired: 1 out]
                n206 = Increment(x=w241) -> (x+1=w259:i32)
                n207 = Greater Or Equal?(x=w259, y=w258) -> (x >= y?=w235:bool)
                n208 = Index Array(array=w238, index=0 ("索引")) -> (element=w248:i32)
                n209 = Index Array(array=w238, index=2 ("索引")) -> (element=w253:i32)
                n210 = Index Array(array=w238, index=1 ("索引")) -> (element=w247:i32)
                n211 = Index Array(array=w238, index=3 ("索引")) -> (element=w252:i32)
                n212 = Number To Decimal String(number=w259) -> (decimal integer string=w244:string)  [unwired: 1 in]
                n213 = Build Array(w248, w247, w253, w252) -> (w231:i32[])
                n214 = call "IMAQ Draw"("Draw Mode"=w250, "Shape to draw"=w243, "Pixel Color"=sgl 0.0, "Coordinates"=w231, "Image Dst"=w236, "Image Src"=w237) -> ("Image Dst Out"=w249:T2)  [unwired: 4 in, 1 out]
                n215 = Concatenate Strings(w244, "#" ("字符串")) -> (w242:string)
                n216 = local read "自定义字体"() -> (w233:T1)
                n217 = Build Array(w248, w247) -> (w234:i32[])
                n218 = call "IMAQ Draw Text"("String"=w242, "Insertion Point"=w234, "Color"=w246, "Font, Size & Style"=w233, "Image Dst"=w236, "Image Src"=w249) -> ("Image Dst Out"=w232:T2)  [unwired: 2 in, 3 out]
                n219 = local write "标注图ROI2Mask"(w232) -> ()
              }
            }
          }
          n220 = local write "穿透图"(w208) -> ()
          n221 = local write "反射图"(w207) -> ()
          n222 = local read "stop"() -> (w203:bool)
          n223 = Or(x=w203, y=w201) -> (x .or. y?=w204:bool)
          n224 = call <vilib>:"Application Directory.vi"() -> ()  [unwired: 1 out]
        }
      }
      event "查看标注": Value Change {
        # "查看指定框的详细信息，包括灰度和面积阈值分割后的结果，提取到的长宽面积等信息"
        n225 = event-data() -> ()  [unwired: 1 in, 6 out]
        n226 = local read "部位信息"() -> (w382:string[])
        n227 = local read "反射图原始路径"() -> (w380:path)
        n228 = local read "穿透图原始路径"() -> (w381:path)
        n229 = local read "产品规格"() -> (w383:cluster{"产品长度（周长）（mm）":dbl, "产品宽度（母线长）（mm）":dbl})
        n230 = local read "灰度阈值"() -> (w384:dbl)
        n231 = local read "框组"() -> (w379:T3)
        n232 = call "输入选择框号"() -> ("框号"=w386:dbl, "确定"=w385:bool)  [unwired: 17 in, 1 out]
        n233 = case shown="真" w385 {
          tunnel: w386 -> [_ w395]
          tunnel: w384 -> [_ w394]
          tunnel: w383 -> [_ w393]
          tunnel: w382 -> [_ w390]
          tunnel: w381 -> [_ w389]
          tunnel: w380 -> [_ w388]
          tunnel: w379 -> [_ w387]
          frame False {
            # "用户取消操作"
          }
          frame True {
            n234 = call "子界面-查看某框和报告生成-第2版.vi"("框号"=w395, "框组"=w387, "反射图原始路径"=w388, "预先配置的灰度阈值"=w394, "穿透图原始路径"=w389, "部位信息"=w390, "产品规格"=w393) -> ("弥散类检测结果"=→"弥散类检测结果":string[][], "分层类检测结果"=→"分层类检测结果":string[][])  [unwired: 11 in]
          }
        }
      }
      event "生成评定结果": Value Change {
        # "最终检测结果全部合并 导入word中"
        # "相当于“查看标注”一栏中的操作做循环，遍历所有框，\n将输出结果叠加为数组，作为最终结果输出并导入word"
        n235 = event-data() -> ()  [unwired: 1 in, 6 out]
        n236 = local read "弥散类检测结果合并"() -> (w402:string[][])
        n237 = local read "分层类检测结果合并"() -> (w403:string[][])
        n238 = local read "穿透图原始路径"() -> (w405:path)
        n239 = local read "反射图原始路径"() -> (w404:path)
        n240 = local read "灰度阈值"() -> (w408:dbl)
        n241 = local read "部位信息"() -> (w407:string[])
        n242 = local read "框组"() -> (w409:T3)
        n243 = local read "产品规格"() -> (w406:cluster{"产品长度（周长）（mm）":dbl, "产品宽度（母线长）（mm）":dbl})
        n244 = local read "框数"() -> (w410:dbl)
        n245 = for {
          N: w410 -> [w468]
          tunnel: w409 -> [w469]
          tunnel: w408 -> [w467]
          tunnel: w407 -> [w466]
          tunnel: w406 -> [w465]
          tunnel: w405 -> [w464]
          tunnel: w404 -> [w463]
          tunnel: w403 -> [w462]
          tunnel: w402 -> [w461]
          tunnel: [w459] -> w401
          tunnel: [w457] -> w399
          n246 = call "子界面-查看某框和报告生成-第2版-不显示界面.vi"("框号"=w468, "框组"=w469, "反射图原始路径"=w463, "预先配置的灰度阈值"=w467, "穿透图原始路径"=w464, "部位信息"=w466, "产品规格"=w465) -> ("弥散类检测结果"=w458:string[][], "分层类检测结果"=w460:string[][])  [unwired: 11 in]
          n247 = Insert Into Array(array=w462, new element=w460) -> (w459:string[][])  [unwired: 2 in]
          n248 = Insert Into Array(array=w461, new element=w458) -> (w457:string[][])  [unwired: 2 in]
        }
        n249 = local write "弥散类检测结果合并"(w399) -> ()
        n250 = local write "分层类检测结果合并"(w401) -> ()
        n251 = flat-sequence {
          tunnel: w401 -> [w415]
          tunnel: w399 -> [w414]
          tunnel: [w414] -> w400
          tunnel: [w413] -> w398
          tunnel: [w412] -> w397
          tunnel: w400 -> [w432]
          tunnel: w398 -> [w431]
          tunnel: w397 -> [w430]
          tunnel: [w455] -> w396
          frame #0 {
            n252 = call <vilib>:"Create Report.vi"("window state (normal)"=T10."no change", "report type"=Report_Type."Word") -> ("report out"=w427:refnum<class "NI_report.lvclass">, "error out"=w423:errorcluster)  [unwired: 12 in]
            n253 = call <vilib>:"Word Easy Title.vi"("report in"=w427, "title"="缺陷评定结果", "font"=T9 {"font name"="", "font size"=18.0, "bold"=1, "italic"=0, "underline"=0, "strike through"=0, "font color"=16777216}, "error in (no error)"=w423) -> ("report out"=w417:refnum<class "NI_report.lvclass">, "error out"=w422:errorcluster)  [unwired: 9 in, 1 out]
            n254 = call <vilib>:"Word Easy Text.vi"("report in"=w417, "text"="分层类", "alignment (left)"=enum16{"Left", "Centered", "Right", "Justify"}."Left", "font"=T9 {"font name"="", "font size"=0.0, "bold"=0, "italic"=0, "underline"=0, "strike through"=0, "font color"=16777216}, "error in (no error)"=w422) -> ("report out"=w418:refnum<class "NI_report.lvclass">, "error out"=w419:errorcluster)  [unwired: 8 in, 1 out]
            n255 = call-poly <vilib>:"Word Easy Table.vi"("report in"=w418, "column headers"=string[] ["框号", "长/mm", "宽/mm", "面积/mm2", "Z值", "部位", "类型", "合格性"], "data"=w415, "error in (no error)"=w419) -> ("report out"=w413:refnum<class "NI_report.lvclass">, "error out"=w412:errorcluster)  [unwired: 9 in, 1 out]
          }
          frame #1 {
            n256 = call <vilib>:"Word Easy Text.vi"("report in"=w431, "text"="弥散类", "alignment (left)"=enum16{"Left", "Centered", "Right", "Justify"}."Left", "font"=T9 {"font name"="", "font size"=0.0, "bold"=0, "italic"=0, "underline"=0, "strike through"=0, "font color"=16777216}, "error in (no error)"=w430) -> ("report out"=w439:refnum<class "NI_report.lvclass">, "error out"=w440:errorcluster)  [unwired: 8 in, 1 out]
            n257 = call-poly <vilib>:"Word Easy Table.vi"("report in"=w439, "column headers"=string[] ["框号", "长/mm", "宽/mm", "面积/mm2", "Z值", "部位", "类型", "合格性"], "data"=w432, "error in (no error)"=w440) -> ("report out"=w438:refnum<class "NI_report.lvclass">, "error out"=w434:errorcluster)  [unwired: 9 in, 1 out]
            n258 = Current VI's Path() -> (path=w446:path)
            n259 = Strip Path(path=w446) -> (stripped path=w445:path)  [unwired: 1 out]
            n260 = Build Path(base path=w445, name or relative path="报表文件.docx" ("名称或相对路径")) -> (appended path=w437:path)
            n261 = call-dynamic "Save Report to File.vi"("report in"=w438, "report file path"=w437, "error in (no error)"=w434) -> ("report out"=w436:refnum<class "NI_report.lvclass">, "error out"=w435:errorcluster)  [unwired: 11 in]
            n262 = call-dynamic "Dispose Report.vi"("report in"=w436, "error in (no error)"=w435) -> ()  [unwired: 13 in, 1 out]
          }
          frame #2 {
            n263 = local read "标注图ROI2Mask"() -> (w447:T2)
            n264 = call <vilib>:"Application Directory.vi"() -> ("Application Directory"=w453:path)
            n265 = Concatenate Strings("_" ("字符串"), ".bmp" ("名称或相对路径")) -> (w452:string)
            n266 = Build Path(base path=w453, name or relative path="database\\" ("名称或相对路径")) -> (appended path=w454:path)
            n267 = Build Path(base path=w454, name or relative path=w452) -> (appended path=w449:path)
            "标注后的图片路径" <- w449
            n268 = call-poly "IMAQ Write File 2"("File Path"=w449, "Image"=w447) -> ()  [unwired: 8 in, 2 out]
          }
          frame #3 {
            n269 = One Button Dialog(message="完成评定并退出程序！\n请查看word报告" ("消息")) -> (true=w455:bool)  [unwired: 1 in]
          }
        }
      }
      event "stop": Value Change {
        # "退出软件"
        n270 = event-data() -> ("NewVal"=w472:bool)  [unwired: 1 in, 4 out]
        n271 = Two Button Dialog(message="是否关闭本软件？" ("消息")) -> (T button?=w474:bool)  [unwired: 2 in]
        n272 = And(x=w472, y=w474) -> (x .and. y?=w471:bool)
        n273 = case shown="真" w471 {
          frame False {
          }
          frame True {
            w475 = TRUE ("All Images? (No)")
            n274 = local read "穿透图"() -> (w477:T2)
            n275 = local read "反射图"() -> (w476:T2)
            n276 = call "IMAQ Dispose"("All Images? (No)"=w475, "Image"=w477) -> ()  [unwired: 4 in, 1 out]
            n277 = call "IMAQ Dispose"("All Images? (No)"=w475, "Image"=w476) -> ()  [unwired: 4 in, 1 out]
            n278 = disable-structure shown="RUN_TIME_ENGINE==True" {
              frame condition #0 {
                n279 = Quit LabVIEW() -> ()  [unwired: 1 in]
              }
              frame condition #1 (active) {
                n280 = Stop() -> ()  [unwired: 1 in]
              }
            }
          }
        }
      }
    }
  }
  "框组" <- T3 [] ("框组")
  "框数" <- 0.0 ("框数")
  "自定义字体" <- T1 {"Desired Font (Application)"=enum."User-specified Font", "[User-specified Font]"={"Font Name"="", "Size"=80, "Strikeout?"=FALSE, "Italic?"=FALSE, "Underline?"=FALSE, "Outline?"=FALSE, "Shadow?"=FALSE, "Bold?"=TRUE, "Rotation Angle"=0.0}, "Horizontal Alignment"=0, "Vertical Alignment"=0} ("Font, Size & Style")
  "部位信息" <- string[] ["", "", "", "", "", "", "", "", ""] ("部位信息")
  "分层类检测结果合并" <- string[][] [] ("弥散类检测结果合并")
  "弥散类检测结果合并" <- string[][] [] ("弥散类检测结果合并")
